vi "Set_VI_Page_Margins.vi"(2 "error in (no error)":errorcluster, 3 "margins":T1={"override VI margins (false)"=FALSE, "margins (1.00)"={"top"=1.0, "left"=1.0, "right"=1.0, "bottom"=1.0}, "measurement system (default)"=0} {"measurement system (default)" items=["Default", "US", "Metric"]; "margins (1.00)"."right" format="%.2f"; "margins (1.00)"."bottom" format="%.2f"; "margins (1.00)"."top" format="%.2f"; "margins (1.00)"."left" format="%.2f"}, 4 "VI Refnum":refnum<vi>) -> (0 "error out":errorcluster, 1 "VI Refnum out":refnum<vi>)   [LabVIEW 2020, in "NI_ReportGenerationCore.lvlib"]
uses:
  <vilib>/Utility/NIReport.llb/NI_ReportGenerationCore.lvlib
  <vilib>/printing/EasyPrintingControls.llb/margins.ctl
  <vilib>/printing/EasyPrintingControls.llb/margin_values.ctl
  <vilib>/printing/EasyPrintingControls.llb/measurement_system.ctl
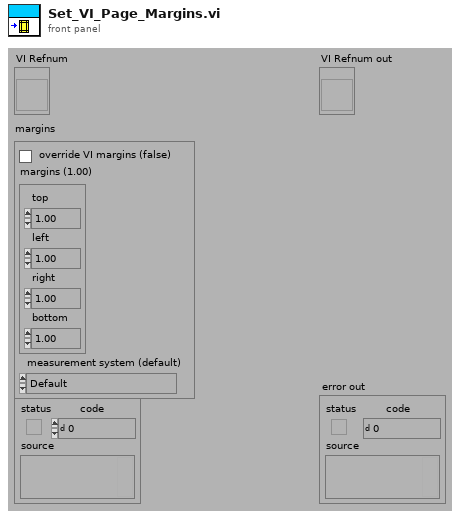
[diagram p1: front panel]
types:
  T1 = typedef "NI_ReportGenerationCore.lvlib/margins.ctl" = cluster{"override VI margins (false)":bool, "margins (1.00)":T2, "measurement system (default)":T3}
  T2 = typedef "NI_ReportGenerationCore.lvlib/margin_values.ctl" = cluster{"top":dbl, "left":dbl, "right":dbl, "bottom":dbl}
  T3 = typedef "NI_ReportGenerationCore.lvlib/measurement_system.ctl" = u16
  T4 = cluster{"top":sgl, "left":sgl, "bottom":sgl, "right":sgl, "measurement system":enum8{"Inches", "cm"}}
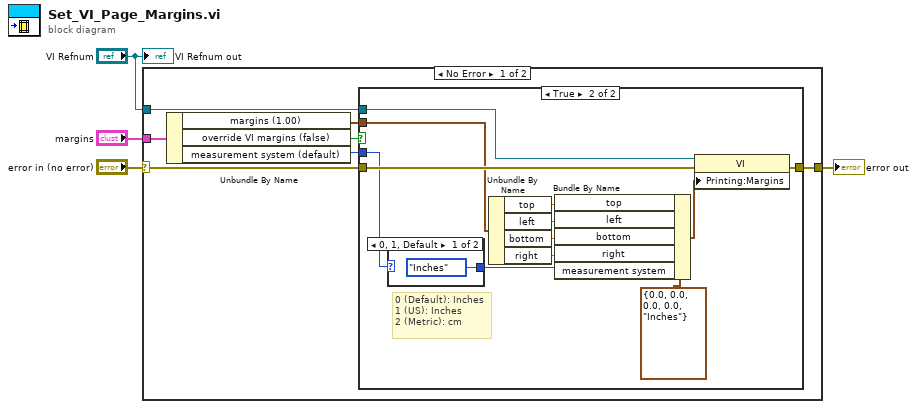
[diagram p0: block diagram]
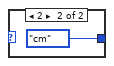
[diagram p3: hidden frame]
diagram:
  n1 = case shown="No Error" "error in (no error)" {
    selector: "error in (no error)" -> [w7 w27]
    tunnel: [w11 w27] -> w4
    tunnel: "margins" -> [w9 _]
    tunnel: "VI Refnum" -> [w8 _]
    frame No Error {
      n2 = Unbundle By Name(w9) -> ("margins (1.00)"=w6:T2, "override VI margins (false)"=w10:bool, "measurement system (default)"=w5:T3)
      n3 = case shown="True" w10 {
        tunnel: w8 -> [_ w22]
        tunnel: w7 -> [w12 w24]
        tunnel: [w12 w23] -> w11
        tunnel: w6 -> [_ w17]
        tunnel: w5 -> [_ w14]
        frame False {
          # "Do not change this setting"
        }
        frame True {
          # "0 (Default): Inches\n1 (US): Inches\n2 (Metric): cm"
          n4 = case shown="0, 1, Default" w14 {
            tunnel: [enum8{"Inches", "cm"}."Inches" ("measurement system") enum8{"Inches", "cm"}."cm" ("measurement system")] -> w13
            frame 0, 1, Default {
            }
            frame 2 {
            }
          }
          n5 = Unbundle By Name(w17) -> ("top"=w21:dbl, "left"=w20:dbl, "bottom"=w19:dbl, "right"=w18:dbl)
          n6 = Bundle By Name(cluster=T4 {"top"=0.0, "left"=0.0, "bottom"=0.0, "right"=0.0, "measurement system"=enum."Inches"} ("Printing:Margins"), "top"=w21, "left"=w20, "bottom"=w19, "right"=w18, "measurement system"=w13) -> (w15:T4)
          n7 = property class="VI"(reference=w22, error in=w24, "Printing:Margins"=w15) -> (error out=w23:errorcluster)  [unwired: 1 out]
        }
      }
    }
    frame Error {
    }
  }
  "error out" <- w4
  "VI Refnum out" <- "VI Refnum"
